vi "Change FP Items Properties.vi"(8 "error in (no error)":errorcluster, 10 "Input + Output":T1, 11 "VI in":refnum<vi>) -> (0 "error out":errorcluster, 3 "VI out":refnum<vi>)   [LabVIEW 2020, in "DocTool.lvlib"]
uses:
  DocTool.lvlib
  TDefs/FP Items Properties.ctl
  TDefs/FP Item Properties.ctl
  TDefs/CopyTag.ctl
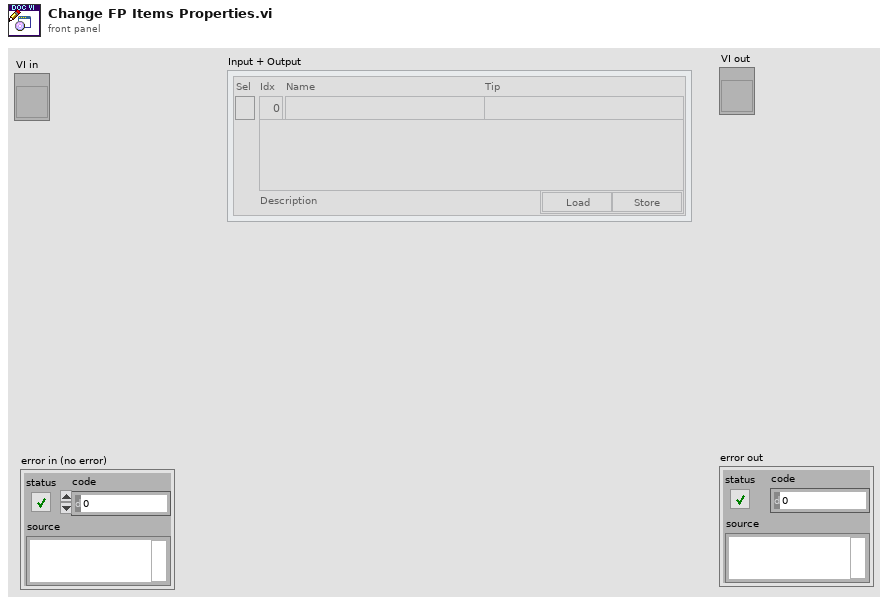
[diagram p1: front panel]
types:
  T1 = typedef "DocTool.lvlib/FP Items Properties.ctl" = T2[]
  T2 = typedef "DocTool.lvlib/FP Item Properties.ctl" = cluster{"Sel":bool, "Idx":i32, "Name":string, "Description":string, "Tip":string, "Load Store":T3}
  T3 = typedef "DocTool.lvlib/CopyTag.ctl" = cluster{"Load":bool, "Store":bool}
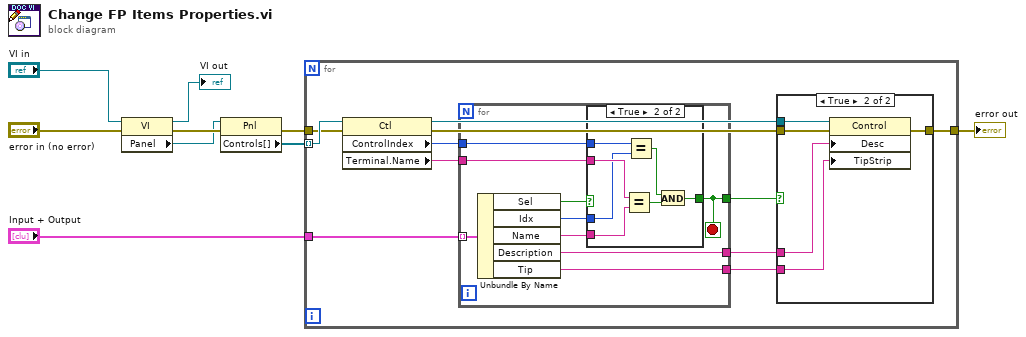
[diagram p0: block diagram]
diagram:
  n1 = property class="VI"(reference="VI in", error in="error in (no error)") -> (reference out=→"VI out":refnum<vi>, error out=w5:errorcluster, "Panel"=w2:refnum<vi>)
  n2 = property class="Pnl"(reference=w2, error in=w5) -> (error out=w4:errorcluster, "Controls[]"=w3:refnum<vi>[])  [unwired: 1 out]
  n3 = for {
    tunnel: w3 -> [w16] mode=indexing
    tunnel: w4 -> [w15]
    tunnel: [w20] -> w9
    tunnel: "Input + Output" -> [w12]
    n4 = property class="Ctl"(reference=w16, error in=w15) -> (reference out=w17:refnum<vi>, error out=w18:errorcluster, "ControlIndex"=w14:i32, "Terminal.Name"=w13:string)
    n5 = for {
      tunnel: w13 -> [w28]
      tunnel: w14 -> [w29]
      tunnel: [w27] -> w19
      tunnel: w12 -> [w26] mode=indexing
      tunnel: [w25] -> w11
      tunnel: [w22] -> w10
      stop <- w27 stop-if-true
      n6 = Unbundle By Name(w26) -> ("Sel"=w21:bool, "Idx"=w24:i32, "Name"=w23:string, "Description"=w22:string, "Tip"=w25:string)
      n7 = case shown="True" w21 {
        tunnel: w29 -> [_ w36]
        tunnel: w28 -> [_ w35]
        tunnel: [_ w32] -> w27
        tunnel: w24 -> [_ w31]
        tunnel: w23 -> [_ w30]
        frame False {
        }
        frame True {
          n8 = Equal?(x=w35, y=w30) -> (x = y?=w33:bool)
          n9 = Equal?(x=w36, y=w31) -> (x = y?=w34:bool)
          n10 = And(x=w34, y=w33) -> (x .and. y?=w32:bool)
        }
      }
    }
    n11 = case shown="True" w19 {
      tunnel: w17 -> [_ w42]
      tunnel: w11 -> [_ w39]
      tunnel: w10 -> [_ w38]
      tunnel: w18 -> [w37 w41]
      tunnel: [w37 w40] -> w20
      frame False {
      }
      frame True {
        n12 = property class="Control"(reference=w42, error in=w41, "Desc"=w38, "TipStrip"=w39) -> (error out=w40:errorcluster)  [unwired: 1 out]
      }
    }
  }
  "error out" <- w9
